vi "Act system PC main.vi"() -> ()   [LabVIEW 2014]
uses:
  <vilib>/Utility/inputDevices.llb/keyboardAcquire.vi
  <vilib>/Utility/inputDevices.llb/closeKeyboard.vi
panel:
  in  "Control Selector":bool
  in  "stop":bool
  out "ServoKeyboard":dbl min=-45.0 max=45.0 step=1.0
  out "PropmotorKeybd":dbl min=-9.0 max=9.0 step=1.0
  out "RT Blink":bool
  out "error IO":errorcluster
  out "PC running":bool
  # "Potentiometer"
  # "Use the arrow keys and the \"/\"\nthe change the values"
  # "Keyboard"
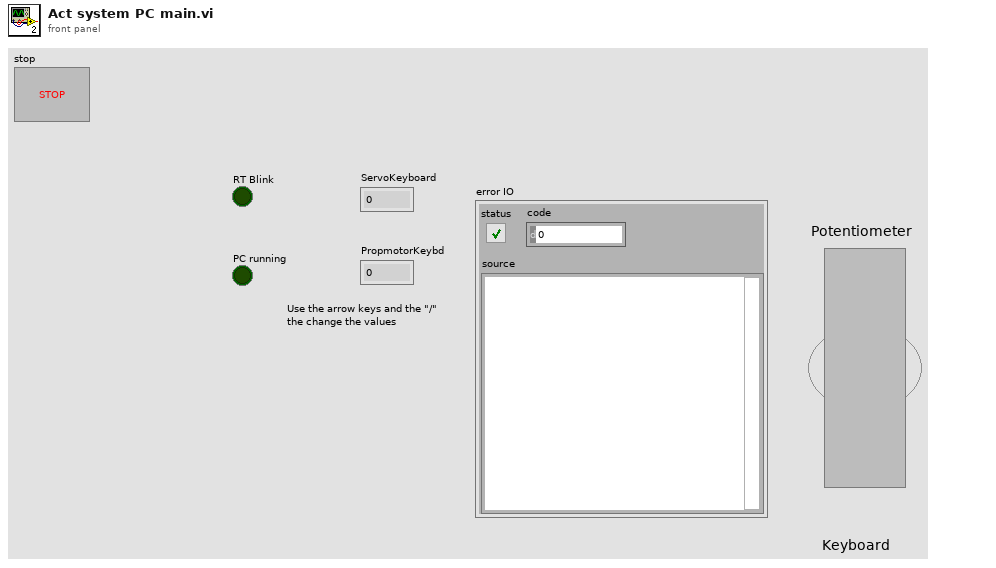
[diagram p1: front panel]
types:
  T1 = enum16{"0", "1", "2", "3", "4", "5", "6", "7", "8", "9", "A", "B", "C", "D", "E", "F", "G", "H", "I", "J", "K", "L", "M", "N", "O", "P", "Q", "R", "S", "T", "U", "V", "W", "X", "Y", "Z", "F1", "F2", "F3", "F4", "F5", "F6", "F7", "F8", "F9", "F10", "F11", "F12", "F13", "F14", "F15", "ADD", "BACK", "BACKSLASH", "CAPITAL", "COMMA", "DECIMAL", "DELETE", "DIVIDE", "DOWN", "END", "EQUALS", "ESCAPE", "GRAVE (`)", "HOME", "INSERT", "LBRACKET", "LCONTROL", "LEFT", "L ALT", "LSHIFT", "LWIN", "MINUS", "MULTIPLY", "NEXT", "NUMLOCK", "NUMPAD_0", "NUMPAD_1", "NUMPAD_2", "NUMPAD_3", "NUMPAD_4", "NUMPAD_5", "NUMPAD_6", "NUMPAD_7", "NUMPAD_8", "NUMPAD_9", "PAUSE", "PERIOD", "PRIOR (PG UP)", "RBRACKET", "RCONTROL", "RETURN", "RIGHT", "R ALT", "RSHIFT", "RWIN", "SCROLL", "SEMICOLON", "SLASH", "SPACE", "SUBTRACT", "TAB", "UP", "ENTER (num pad)", "' (quote)"}[]
  T2 = enum16{"0", "1", "2", "3", "4", "5", "6", "7", "8", "9", "A", "B", "C", "D", "E", "F", "G", "H", "I", "J", "K", "L", "M", "N", "O", "P", "Q", "R", "S", "T", "U", "V", "W", "X", "Y", "Z", "F1", "F2", "F3", "F4", "F5", "F6", "F7", "F8", "F9", "F10", "F11", "F12", "F13", "F14", "F15", "ADD", "BACK", "BACKSLASH", "CAPITAL", "COMMA", "DECIMAL", "DELETE", "DIVIDE", "DOWN", "END", "EQUALS", "ESCAPE", "GRAVE (`)", "HOME", "INSERT", "LBRACKET", "LCONTROL", "LEFT", "L ALT", "LSHIFT", "LWIN", "MINUS", "MULTIPLY", "NEXT", "NUMLOCK", "NUMPAD_0", "NUMPAD_1", "NUMPAD_2", "NUMPAD_3", "NUMPAD_4", "NUMPAD_5", "NUMPAD_6", "NUMPAD_7", "NUMPAD_8", "NUMPAD_9", "PAUSE", "PERIOD", "PRIOR (PG UP)", "RBRACKET", "RCONTROL", "RETURN", "RIGHT", "R ALT", "RSHIFT", "RWIN", "SCROLL", "SEMICOLON", "SLASH", "SPACE", "SUBTRACT", "TAB", "UP", "ENTER (num pad)", "' (quote)"}
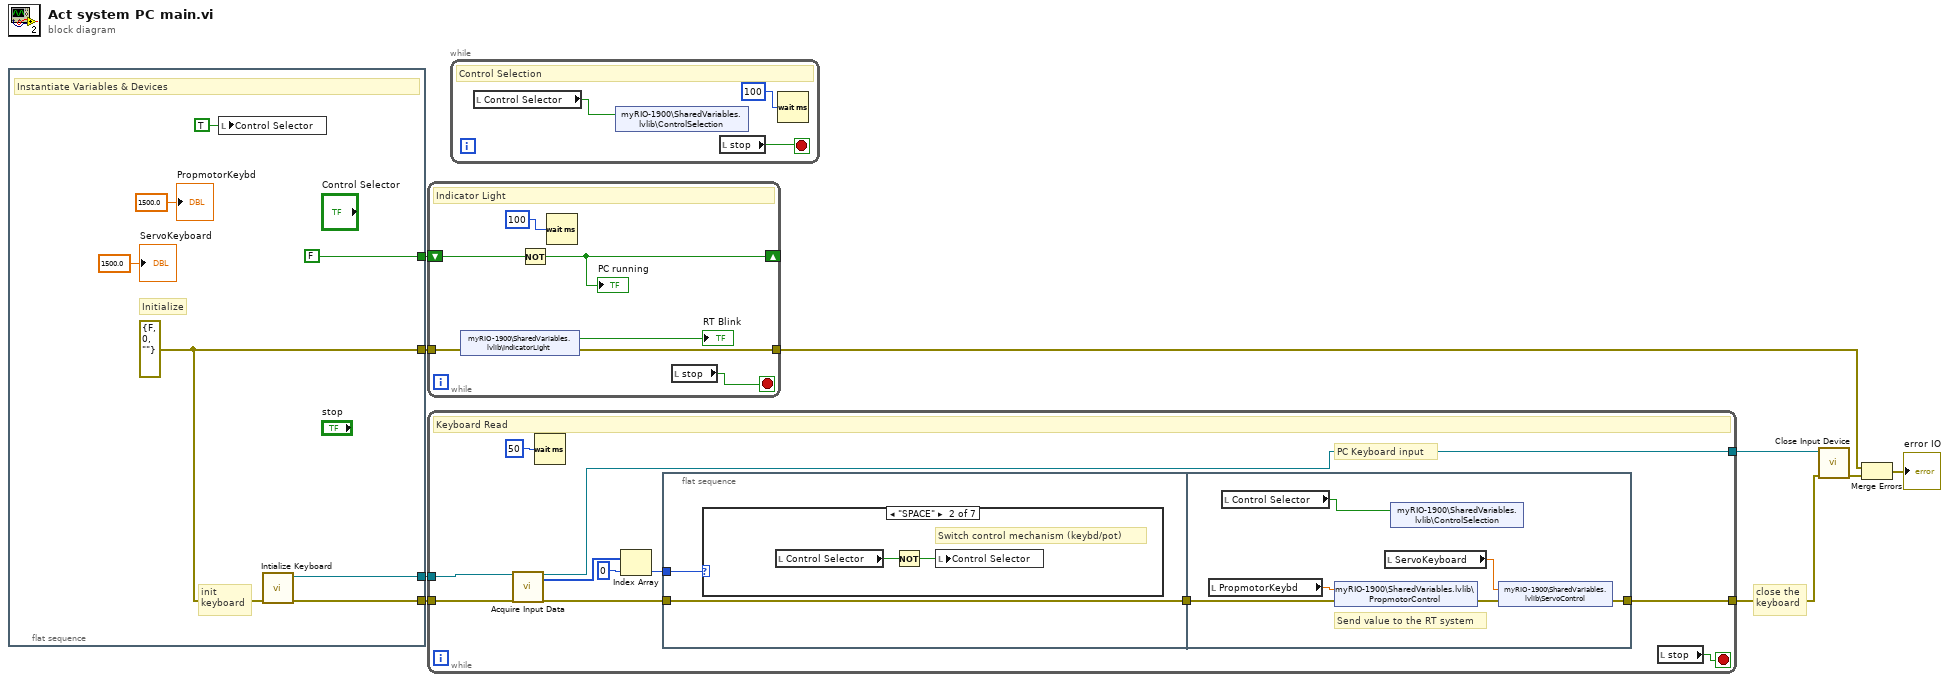
[diagram p0: block diagram]
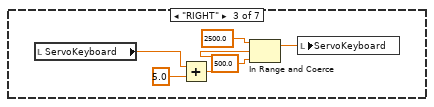
[diagram p3: hidden frame]
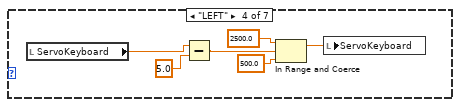
[diagram p4: hidden frame]
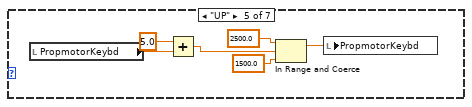
[diagram p5: hidden frame]
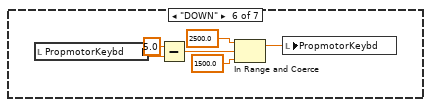
[diagram p6: hidden frame]
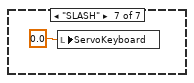
[diagram p7: hidden frame]
diagram:
  # "close the\nkeyboard"
  n1 = flat-sequence {
    tunnel: [w16] -> w8
    tunnel: [w15] -> w9
    tunnel: [w14] -> w7
    tunnel: [FALSE] -> w4
    frame #0 {
      w14 = errorcluster {"status"=FALSE, "code"=0, "source"=""} ("error in (no error)")
      # "Initialize"
      # "init\nkeyboard"
      # "Instantiate Variables & Devices"
      n2 = local write "Control Selector"(TRUE ("Control Selector")) -> ()
      n3 = call <vilib>:"Intialize Keyboard.vi"("error in (no error)"=w14) -> ("error out"=w15:errorcluster, "device ID"=w16:refnum<k1>)  [unwired: 9 in]
      "ServoKeyboard" <- 1500.0 ("ServoKeyboard")
      "PropmotorKeybd" <- 1500.0 ("PropmotorKeybd")
    }
  }
  n4 = while {
    shift-right: [w22] -> _
    shift-left: w4 -> [w23]
    tunnel: w7 -> [w21]
    tunnel: [w20] -> w5
    stop <- w17 stop-if-true
    # "Indicator Light"
    n5 = shared-variable "myRIO-1900\\SharedVariables.lvlib\\IndicatorLight"(error in=w21) -> (→"RT Blink":bool, error out=w20:errorcluster)
    n6 = Not(x=w23) -> (.not. x?=w22:bool)
    "PC running" <- w22
    n7 = Wait (ms)(milliseconds to wait=u32 100) -> ()  [unwired: 1 out]
    n8 = local read "stop"() -> (w17:bool)
  }
  n9 = while {
    tunnel: w9 -> [w32]
    tunnel: w8 -> [w31]
    tunnel: [w25] -> w3
    tunnel: [w24] -> w2
    stop <- w33 stop-if-true
    # "PC Keyboard input"
    # "Keyboard Read"
    n10 = call-poly <vilib>:"Acquire Input Data.vi"("device ID"=w31, "error in (no error)"=w32) -> ("device ID"=w24:refnum<k1>, "keys pressed"=w30:T1, "error out"=w27:errorcluster)  [unwired: 15 in]
    n11 = Wait (ms)(milliseconds to wait=u32 50) -> ()  [unwired: 1 out]
    n12 = Index Array(array=w30, index=0) -> (element=w28:T2)
    n13 = flat-sequence {
      tunnel: w28 -> [w36]
      tunnel: w27 -> [w35]
      tunnel: [w35] -> w26
      tunnel: w26 -> [w68]
      tunnel: [w65] -> w25
      frame #0 {
        n14 = case shown="\"SPACE\"" w36 {
          frame "0", Default {
            # "Do nothing for all the other keys"
          }
          frame "SPACE" {
            # "Switch control mechanism (keybd/pot)"
            n15 = local read "Control Selector"() -> (w37:bool)
            n16 = Not(x=w37) -> (.not. x?=w38:bool)
            n17 = local write "Control Selector"(w38) -> ()
          }
          frame "RIGHT" {
            n18 = local read "ServoKeyboard"() -> (w41:dbl)
            n19 = Add(x=w41, y=5.0) -> (x+y=w40:dbl)
            n20 = In Range and Coerce(upper limit=2500.0, x=w40, lower limit=500.0) -> (coerced(x)=w44:dbl)  [unwired: 1 out]
            n21 = local write "ServoKeyboard"(w44) -> ()
          }
          frame "LEFT" {
            n22 = local read "ServoKeyboard"() -> (w46:dbl)
            n23 = Subtract(x=w46, y=5.0) -> (x-y=w47:dbl)
            n24 = In Range and Coerce(upper limit=2500.0, x=w47, lower limit=500.0) -> (coerced(x)=w48:dbl)  [unwired: 1 out]
            n25 = local write "ServoKeyboard"(w48) -> ()
          }
          frame "UP" {
            n26 = local read "PropmotorKeybd"() -> (w56:dbl)
            n27 = Add(x=5.0, y=w56) -> (x+y=w52:dbl)
            n28 = In Range and Coerce(upper limit=2500.0, x=w52, lower limit=1500.0) -> (coerced(x)=w53:dbl)  [unwired: 1 out]
            n29 = local write "PropmotorKeybd"(w53) -> ()
          }
          frame "DOWN" {
            n30 = local read "PropmotorKeybd"() -> (w62:dbl)
            n31 = Subtract(x=5.0, y=w62) -> (x-y=w59:dbl)
            n32 = In Range and Coerce(upper limit=2500.0, x=w59, lower limit=1500.0) -> (coerced(x)=w58:dbl)  [unwired: 1 out]
            n33 = local write "PropmotorKeybd"(w58) -> ()
          }
          frame "SLASH" {
            n34 = local write "ServoKeyboard"(0.0) -> ()
          }
        }
      }
      frame #1 {
        # "Send value to the RT system"
        n35 = local read "PropmotorKeybd"() -> (w69:dbl)
        n36 = local read "Control Selector"() -> (w64:bool)
        n37 = shared-variable "myRIO-1900\\SharedVariables.lvlib\\PropmotorControl"(w69, error in=w68) -> (error out=w67:errorcluster)
        n38 = local read "ServoKeyboard"() -> (w66:dbl)
        n39 = shared-variable "myRIO-1900\\SharedVariables.lvlib\\ControlSelection"(w64) -> ()  [unwired: 1 in, 1 out]
        n40 = shared-variable "myRIO-1900\\SharedVariables.lvlib\\ServoControl"(w66, error in=w67) -> (error out=w65:errorcluster)
      }
    }
    n41 = local read "stop"() -> (w33:bool)
  }
  n42 = while {
    stop <- w72 stop-if-true
    # "Control Selection"
    n43 = local read "Control Selector"() -> (w70:bool)
    n44 = shared-variable "myRIO-1900\\SharedVariables.lvlib\\ControlSelection"(w70) -> ()  [unwired: 1 in, 1 out]
    n45 = local read "stop"() -> (w72:bool)
    n46 = Wait (ms)(milliseconds to wait=u32 100) -> ()  [unwired: 1 out]
  }
  n47 = call-poly <vilib>:"Close Input Device.vi"("error in (no error)"=w3, "device ID"=w2) -> ("error out"=w1:errorcluster)  [unwired: 8 in]
  n48 = Merge Errors(w5, w1) -> (→"error IO":errorcluster)
